vi "Constructor.vi"(11 "House Blend in":refnum<class "House Blend.lvclass">) -> (3 "House Blend out":refnum<class "House Blend.lvclass">)   [LabVIEW 2011, in "House Blend.lvclass"]
uses:
  House Blend.lvclass
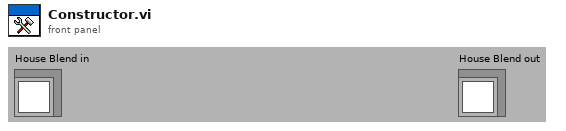
[diagram p1: front panel]
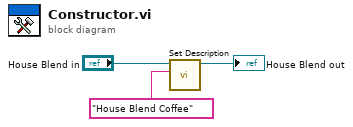
[diagram p0: block diagram]
diagram:
  n1 = call-dynamic "Set Description.vi"("Description"="House Blend Coffee", "Beverage in"="House Blend in") -> ("Beverage out"=→"House Blend out":refnum<class "House Blend.lvclass">)  [unwired: 9 in]
